vi "ZAlign_Modulo_RoundUp.vi"(11 "Value in":i32 caption="Value In") -> (2 "Grid_Size":i32=12, 3 "Value out":i32)   [LabVIEW 2014, in "ZAlign.lvlib"]
doc: "ZAlign.lvlib:ZAlign_Modulo_RoundUp.vi\n----------------------------------------------\nModulo RoundUp\n\nInputs:\n---------------------\n- Value In : I16; \n\nOutputs:\n---------------------\n- Grid_Size : I16; \n- Value out : I16; \n\n----------------------------------------------\n16/03/2015\nZühlke Engineering AG\nCH-8952 Schlieren\nwww.zuehlke.com"
uses:
  ZAlign.lvlib
  <vilib>/Utility/config.llb/NI_LVConfig.lvlib
  <vilib>/Utility/config.llb/Read Key (I32).vi
panel:
  # "Connector Pane"
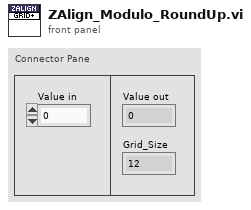
[diagram p1: front panel]
types:
  T1 = typedef "NI_LVConfig.lvlib/Config Data RefNum.ctl" = refnum<k1>
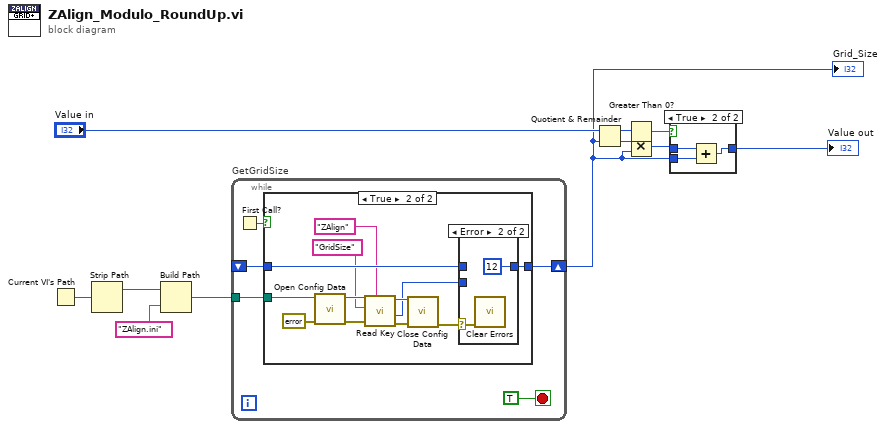
[diagram p0: block diagram]
diagram:
  n1 = Current VI's Path() -> (path=w4:path)
  n2 = Strip Path(path=w4) -> (stripped path=w3:path)  [unwired: 1 out]
  n3 = Build Path(base path=w3, name or relative path="ZAlign.ini") -> (appended path=w1:path)
  n4 = while "GetGridSize" {
    shift-right: [w13] -> w5
    shift-left: _ -> [w12]
    tunnel: w1 -> [w14]
    stop <- TRUE stop-if-true
    n5 = First Call?() -> (First Call?: T/F=w15:bool)
    n6 = case shown="True" w15 {
      tunnel: w14 -> [_ w24]
      tunnel: [w17 w21] -> w13
      tunnel: w12 -> [w17 w20]
      frame False {
      }
      frame True {
        n7 = call <vilib>:"Open Config Data.vi"("error in (no error)"=errorcluster {"status"=FALSE, "code"=0, "source"=""}, "configuration file path"=w24) -> ("error out"=w29:errorcluster, "refnum"=w28:T1)  [unwired: 7 in, 1 out]
        n8 = call-poly <vilib>:"Read Key.vi"("section"="ZAlign", "error in (no error)"=w29, "key"="GridSize" ("section"), "refnum"=w28) -> ("error out"=w27:errorcluster, "value"=w22:i32, "refnum out"=w26:T1)  [unwired: 4 in, 1 out]
        n9 = call <vilib>:"Close Config Data.vi"("error in (no error)"=w27, "refnum"=w26) -> ("error out"=w23:errorcluster)  [unwired: 8 in, 1 out]
        n10 = case shown="Error" w23 {
          selector: w23 -> [_ w32]
          tunnel: w22 -> [w30 _]
          tunnel: [w30 12 ("y")] -> w21
          tunnel: w20 -> [_ _]
          frame No Error {
          }
          frame Error {
            n11 = call <vilib>:"Clear Errors.vi"("error in (no error)"=w32) -> ()  [unwired: 5 in, 2 out]
          }
        }
      }
    }
  }
  "Grid_Size" <- w5
  n12 = Quotient & Remainder(x="Value in", y=w5) -> (x-y*floor(x/y)=w9:i32, floor(x/y)=w7:i32)
  n13 = Greater Than 0?(x=w9) -> (x > 0?=w10:bool)
  n14 = Multiply(x=w7, y=w5) -> (x*y=w6:i32)
  n15 = case shown="True" w10 {
    tunnel: w6 -> [w33 w36]
    tunnel: w5 -> [_ w35]
    tunnel: [w33 w34] -> w11
    frame False {
    }
    frame True {
      n16 = Add(x=w36, y=w35) -> (x+y=w34:i32)
    }
  }
  "Value out" <- w11
